vi "Get Multicast Config.vi"(8 "error in (no error)":errorcluster, 11 "Group Config in":refnum<class "Group Config.lvclass">) -> (0 "error out":errorcluster, 2 "Multicast Config":T1, 3 "Group Config out":refnum<class "Group Config.lvclass">)   [LabVIEW 2020, in "VectoConfig.lvlib" / "Group Config.lvclass"]
uses:
  Group Config.lvclass
  Publish Config.ctl
  Group Config.lvclass/Group Config.ctl
  VectoConfig/VectoConfig.lvlib
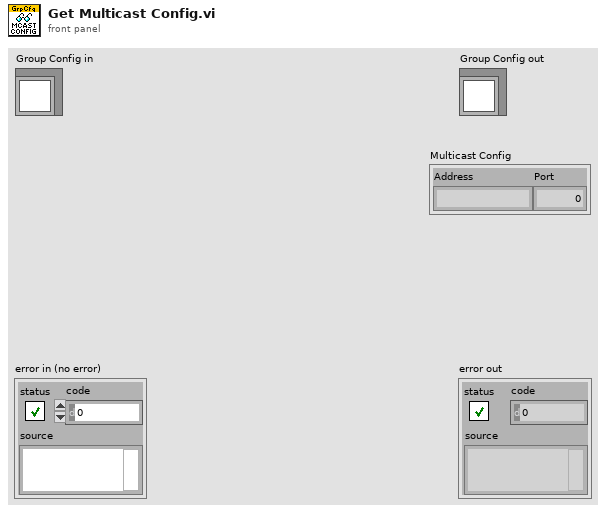
[diagram p1: front panel]
types:
  T1 = typedef "VectoConfig.lvlib/Publish Config.ctl" = cluster{"Address":string, "Port":u16}
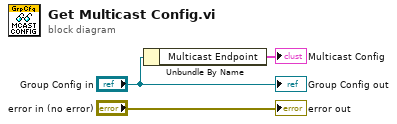
[diagram p0: block diagram]
diagram:
  n1 = Unbundle By Name("Group Config in") -> ("Multicast Endpoint"=→"Multicast Config":T1)
  "error out" <- "error in (no error)"
  "Group Config out" <- "Group Config in"
